vi "ComputeIndentation.vi"(11 "MsgSerializer in":refnum<class "MsgSerializer.lvclass">) -> (2 "indentation":string)   [LabVIEW 2013, in "Caraya.lvlib" / "MsgSerializer.lvclass"]
uses:
  MsgSerializer.lvclass
  MsgSerializer.lvclass/MsgSerializer.ctl
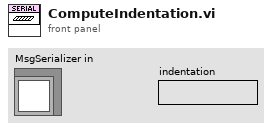
[diagram p1: front panel]
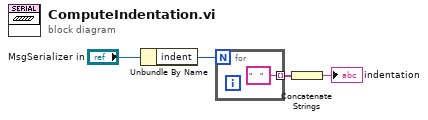
[diagram p0: block diagram]
diagram:
  n1 = Unbundle By Name("MsgSerializer in") -> ("indent"=w2:i32)
  n2 = for {
    N: w2 -> [_]
    tunnel: ["    " ("string")] -> w3 mode=indexing
  }
  n3 = Concatenate Strings(w3) -> (→"indentation":string)
